vi "Create E&S emibin file.vi"(0 "file path (use dialog)":path, 11 "error in (no error)":errorcluster, 12 "E&# File type ID(0, generic)":u16, 13 "E&S File type Version(0, Unset)":u8) -> (4 "refnum out":refnum<file>, 15 "error out":errorcluster)   [LabVIEW 2011]
uses:
  <vilib>/Utility/libraryn.llb/Check if File or Folder Exists.vi
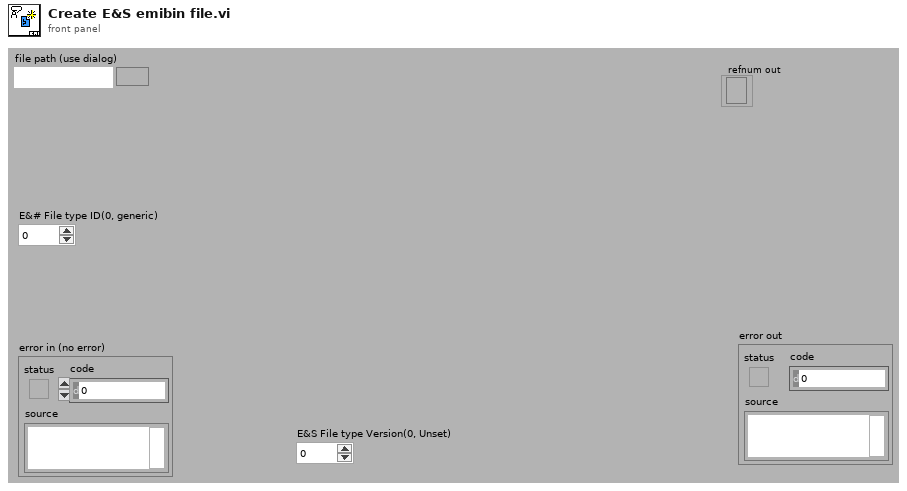
[diagram p1: front panel]
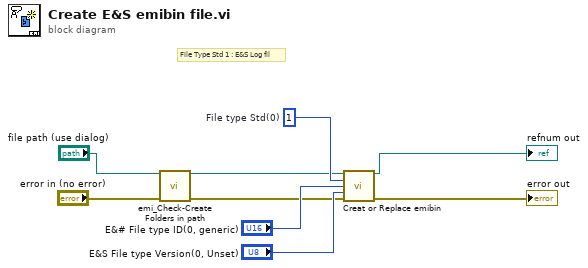
[diagram p0: block diagram]
diagram:
  w7 = u8 1  # File type Std(0)
  # "File Type Std 1 : E&S Log fil"
  n1 = call "emi_Check-Create Folders in path.vi"("Path including file"="file path (use dialog)", "error in (no error)"="error in (no error)") -> ("Path out"=w1:path, "error out"=w3:errorcluster)  [unwired: 11 in, 1 out]
  n2 = call "Creat or Replace emibin.vi"("file path"=w1, "File type Std(0)"=w7, "File type ID"="E&# File type ID(0, generic)", "File type Version"="E&S File type Version(0, Unset)", "error in (no error)"=w3) -> ("refnum out"=→"refnum out":refnum<file>, "error out"=→"error out":errorcluster)  [unwired: 9 in]
